vi "KM_fancytorque.vi"() -> ()   [LabVIEW 2016]
uses:
  plot refs -- filter related.ctl
  KM_ControlHFLIcommand.ctl
  cursor winow.ctl
  cursor window action.ctl
  KM_file -- read-write control.ctl
  MQMUser/Documents/Interfaces/Magnet_August_der_Starke.vi
  circle corners.ctl
  lorentzian.ctl
  KM_SystemParameters.ctl
  <vilib>/event_ctls.llb/eventvkey.ctl
  wavepacket.ctl
  filter method control.ctl
  peak -- parameters -- complex fit.ctl
  parameters -- scan monitor control.ctl
panel:
  out "Array of Refnums":refnum<visa-resource-name>[](array[refnum])=["COM3", "16T-Cryocon", "16T-LevelMeter", "16T-Model4G"]
  in  "Update range":bool
  out "Plot: freq vs T":cluster{dbl[], dbl[]}(graph)={[-100.0], [0.0]}
  in  "scan monitor control":T1={"gamma acc. frac. - min "=0.3, "gamma acc frac.. - max"=3.0, "peak acc. fraction (af)"=5.0, "min peak acc. window (kHz)"=0.5, "use"=enum."fraction", "abs gamma min(kHz)"=0.005, "abs gamma max(kHz)"=5.0, "# points"=5, "gamma-factor (fa)"=12.0, "interpolate"=enum."line", "init"=TRUE, "Unique strike parameters"=TRUE, "max peak acc. window (kHz)"=10.0, "spacing factor"=1.5, "iterate #"=1, "overwrite ctl?"=FALSE, "write _m files?"=FALSE, "max slope (kHz/sweep)"=0.5, "funnel state"=enum."funnel open"}
  in  "Plot frequency shift":bool
  in  "Tab : all plot":enum32{"Page 1"}(tab)
  in  "Save frequency scan":path=path "C:/Data/Kim/FancyTorque/YHerb"
  in  "File name":string="lowT_turnonfield"
  in  "ZI HFLI System Parameters IN":T2={"IP Address"="DEV987", "Start (Hz)"=48440.0, "Stop (Hz)"=48480.0, "Filter Order"=4, "Number of Points"=500, "Precision"=0, "Bandwidth (Hz)"=50.0, "Averaging"=1, "Log Sweep"=FALSE, "Demod"=0} {"Averaging" items=["1"=1, "2"=2, "4"=4, "16"=16, "32"=32, "64"=64]; "Bandwidth (Hz)" format="%#_p"; "Precision" items=["Low", "Med", "High"]; "Number of Points" min=2 max=66000; "Filter Order" items=["6, 1st"=1, "12, 2nd"=2, "18, 3rd"=3, "24, 4th"=4, "30, 5th"=5, "36, 6th"=6, "42, 7th"=7, "48, 8th"=8]; "Stop (Hz)" format="%_5p"; "Start (Hz)" format="%_5p"}
  in  "cursor bracket: All, data window":T3={"left"=48455.25, "right "=48459.75, "center"=48457.5, "window"=4.5, "cursors"=[0, 1, 2], "relative"=0, "absolute"=0, "fixed vertical offset"=0.0, "vertical offset"=0.0, "skew"=0.0, "default window frac"=0.1, "kind"=enum."symmetric", "skew.left"=0.5, "skew.right"=0.5, "Plot ref"=refnum, "wing order"=enum."forw"}
  in  "Update system parameters":bool
  out "Plot: All":cluster{"all rows":dbl[], "all rows":dbl[]}[](graph)
  in  "Tab : everything":T4(tab)
  in  "Tab :  Fit controls":enum32{"complex plane", "complex plane 2"}(tab)
  in  "Plot: fragment - filter":cluster{dbl[], dbl[]}[](graph)=[{[], []}, {[], []}, {[], []}, {[], []}]
  in  "scale gauge: Plot: complex plane - filter":dbl(slide)=0.015780000000000002 min=0.0 max=0.3 step=1e-05 scale=0.0001..0.3 scale format="%#_5g"
  in  "Plot: complex plane - filter":cluster{dbl[], dbl[]}[](graph)=[{[], []}, {[], []}, {[0.0, 0.0, 0.0, 0.0, 0.0, 0.0, 0.0, 0.0, 0.0, 0.0, 0.0, 0.0, 0.0, 0.0, 0.0, 0.0, 0.0, 0.0, 0.0, 0.0, 0.0, 0.0, 0.0, 0.0, 0.0, 0.0, 0.0, 0.0, 0.0, 0.0, 0.0, 0.0, 0.0, 0.0, 0.0, 0.0, 0.0, 0.0, 0.0, 0.0, 0.0, 0.0, 0.0, 0.0, 0.0, 0.0, 0.0, 0.0, 0.0, 0.0, 0.0, 0.0, 0.0, 0.0, 0.0, 0.0, 0.0, 0.0, 0.0, 0.0, 0.0, 0.0, 0.0, 0.0, 0.0, 0.0, 0.0, 0.0, 0.0, 0.0, 0.0, 0.0, 0.0, 0.0, 0.0, 0.0, 0.0, 0.0, 0.0, 0.0, 0.0, 0.0, 0.0, 0.0, 0.0, 0.0, 0.0, 0.0, 0.0, 0.0, 0.0, 0.0, 0.0, 0.0, 0.0, 0.0, 0.0, 0.0, 0.0, 0.0], [0.0, 0.0, 0.0, 0.0, 0.0, 0.0, 0.0, 0.0, 0.0, 0.0, 0.0, 0.0, 0.0, 0.0, 0.0, 0.0, 0.0, 0.0, 0.0, 0.0, 0.0, 0.0, 0.0, 0.0, 0.0, 0.0, 0.0, 0.0, 0.0, 0.0, 0.0, 0.0, 0.0, 0.0, 0.0, 0.0, 0.0, 0.0, 0.0, 0.0, 0.0, 0.0, 0.0, 0.0, 0.0, 0.0, 0.0, 0.0, 0.0, 0.0, 0.0, 0.0, 0.0, 0.0, 0.0, 0.0, 0.0, 0.0, 0.0, 0.0, 0.0, 0.0, 0.0, 0.0, 0.0, 0.0, 0.0, 0.0, 0.0, 0.0, 0.0, 0.0, 0.0, 0.0, 0.0, 0.0, 0.0, 0.0, 0.0, 0.0, 0.0, 0.0, 0.0, 0.0, 0.0, 0.0, 0.0, 0.0, 0.0, 0.0, 0.0, 0.0, 0.0, 0.0, 0.0, 0.0, 0.0, 0.0, 0.0, 0.0]}, {[0.0, 0.0, 0.0], [0.0, 0.0, 0.0]}, {[nan, nan, nan, nan, nan, nan, nan, nan, nan, nan, nan, nan, nan, nan, nan, nan, nan, nan, nan, nan], [nan, nan, nan, nan, nan, nan, nan, nan, nan, nan, nan, nan, nan, nan, nan, nan, nan, nan, nan, nan]}, {[0.0, 0.0, 0.0, 0.0, 0.0, 0.0, 0.0, 0.0, 0.0, 0.0, 0.0, 0.0, 0.0, 0.0, 0.0, 0.0, 0.0, 0.0, 0.0, 0.0], [0.0, 0.0, 0.0, 0.0, 0.0, 0.0, 0.0, 0.0, 0.0, 0.0, 0.0, 0.0, 0.0, 0.0, 0.0, 0.0, 0.0, 0.0, 0.0, 0.0]}]
  out "Plot: dz/domega":cluster{"omega out":dbl[], dbl[]}(graph)
  out "Plot: win omega":T5(graph)
  out "Plot: phase":cluster{"omega out":dbl[], dbl[]}(graph)
  out "Plot: phase around center":cluster{dbl[], dbl[]}[](graph)
  out "Plot: fragment":cluster{dbl[], dbl[]}[](graph)
  out "Plot: complex plane":cluster{dbl[], dbl[]}[](graph)=[{[], []}, {[nan, nan, nan, nan, nan, nan, nan, nan, nan, nan, nan, nan, nan, nan, nan, nan, nan, nan, nan, nan, nan, nan, nan, nan, nan, nan, nan, nan, nan, nan, nan, nan, nan, nan, nan, nan, nan, nan, nan, nan, nan, nan, nan, nan, nan, nan, nan, nan, nan, nan], [nan, nan, nan, nan, nan, nan, nan, nan, nan, nan, nan, nan, nan, nan, nan, nan, nan, nan, nan, nan, nan, nan, nan, nan, nan, nan, nan, nan, nan, nan, nan, nan, nan, nan, nan, nan, nan, nan, nan, nan, nan, nan, nan, nan, nan, nan, nan, nan, nan, nan]}, {[nan, nan, nan, nan, nan, nan, nan, nan, nan, nan, nan, nan, nan, nan, nan, nan, nan, nan, nan, nan], [nan, nan, nan, nan, nan, nan, nan, nan, nan, nan, nan, nan, nan, nan, nan, nan, nan, nan, nan, nan]}, {[nan, nan, nan, nan, nan, nan, nan, nan, nan, nan, nan, nan, nan, nan, nan, nan, nan, nan, nan, nan], [nan, nan, nan, nan, nan, nan, nan, nan, nan, nan, nan, nan, nan, nan, nan, nan, nan, nan, nan, nan]}, {[nan, nan, nan, nan, nan, nan, nan, nan, nan, nan, nan, nan, nan, nan, nan, nan, nan, nan, nan, nan], [nan, nan, nan, nan, nan, nan, nan, nan, nan, nan, nan, nan, nan, nan, nan, nan, nan, nan, nan, nan]}, {[nan, nan, nan, nan, nan, nan, nan, nan, nan, nan, nan, nan, nan, nan, nan, nan, nan, nan, nan, nan], [nan, nan, nan, nan, nan, nan, nan, nan, nan, nan, nan, nan, nan, nan, nan, nan, nan, nan, nan, nan]}, {[], []}]
  in  "scale gauge: Plot: complex plane":dbl(slide)=0.013730000000000001 min=0.0 max=0.3 step=1e-05 scale=0.0001..1.0 scale format="%#_2g"
  out "window width (kHz)":dbl=76.27809365793496
  out "window center (kHz)":dbl=3399.029286744401
  out "# of points in window":dbl=953.475933538175
  in  "use fast fit?":bool
  out "pm lorentzian":T6={"Amplitude"=nan, "omega(0)"=0.0, "Gamma"=0.0, "phase"=nan, "Q"=nan, "Norm  Ampl"=nan, "z (inf)"=nan+nani, "4corners"={"z (-pi/2)"=nan+nani, "z(inf)"=nan+nani, "z (pi/2)"=nan+nani, "z center"=nan+nani, "z(0)"=nan+nani, "radius"=nan}} {"z (inf)" format="%#9_9f"; "Q" format="%#9_9f"; "phase" format="%#9_9f"; "Gamma" format="%#9_9f"; "omega(0)" format="%#9_9f"}
  in  "plot staff":enum16{"plot", "do not plot", "a"}(ring)
  in  "Take data":bool=TRUE
  in  "Tab : parameters":enum32{"Page 1"}(tab)
  out "VKey":T8=enum."Return"
  out "Char":i16
  out "Voltage out":cdb[](array[numeric])=[0.0012845876568090215+0.0006495888225572617i, 0.0006617392839354205-0.002163791666582164i, 0.00032146349849778734-0.0008539323430354452i, 0.0007212690079914407-0.0003340132939741794i, 0.0018796838985498537-0.00041382611356276136i, 0.002110516048657634-0.0009455346019583315i, 0.00205017696245498-0.0010893795945051384i, 0.0019478328941950674-0.0014483165844385926i, 0.0018835525878900681-0.001474948715399006i, 0.0013372864726134792-0.0017269565608841629i, 0.0012769136053726307-0.0015682015434732959i, 0.0011465878308944987-0.001449912746741602i, 0.0011207935884417488-0.0014499150090787223i, 0.0012200224050478575-0.001454330158192838i, 0.001088103973473641-0.0013059205845030238i, 0.001072088135514426-0.0012144891963959052i, 0.0011292588329624431-0.0008751147544548225i, 0.0011981393964060746-0.0009880476045942583i, 0.001133057536849098-0.0010263007167294748i, 0.0011273462401748915-0.0011399691730504498i, 0.0012584422806093418-0.0010608947550812256i, 0.0011560305040308565-0.0010341591377315345i, 0.001276567934756488-0.00111907533128109i, 0.0013066630041961857-0.0011064460918718418i, 0.0013770198549916794-0.0010463285175782726i, 0.001314665107953928-0.0009875590410208187i, 0.0013770356718726985-0.0011716715953778503i, 0.0014487115235704165-0.0011144718894301464i, 0.0014447364087279003-0.0012343495924517127i, 0.0014921485718953887-0.0011853078768784987i, 0.0015783944605238338-0.001213834817063661i, 0.0016223257172798958-0.0011418240543088765i, 0.0016368737143736612-0.001111623978754091i, 0.0016204398102554545-0.0010964954268465582i, 0.0016331401454112604-0.0010700307948267869i, 0.0016423618897952804-0.0009410751832895035i, 0.0016255939283663164-0.0009421622662113829i, 0.0016412998435803663-0.0009531512264980333i, 0.0016134375053353611-0.0009005165103711552i, 0.0016054817151254191-0.0009402602111659055i, 0.0015706664673148592-0.0009279919272101116i, 0.0015994002900568897-0.0009699193362076616i, 0.001638610958103286-0.001007835954895566i, 0.001629322361562981-0.0009580956979464267i, 0.0016613871405357136-0.0009785147196610432i, 0.0017233134934095098-0.0009736245027034165i, 0.0016803207109420183-0.0009995146170615366i, 0.0017007833914218493-0.000957625565568956i, 0.0016916365400226811-0.000857954594368348i, 0.0016717789688494263-0.0009179629793560123i, 0.0016734726456965087-0.0009260924684352465i, 0.0017251671295331528-0.000981940013575436i, 0.0017240578858999007-0.0008851005821558551i, 0.001740616055028208-0.0008509351236963866i, 0.0016837038942047505-0.0009158599053328468i, 0.0017068774584739978-0.0008981950544142098i, 0.0017784029248129117-0.0008343945412286558i, 0.0017220291571895204-0.0009102684605824946i, 0.0017414811568882292-0.0008954153399333319i, 0.001791730794309786-0.00086317641219086i, 0.0018095326778530107-0.0008176560683240543i, 0.0018408224973787044-0.0008618058990086667i, 0.001863514774019469-0.0008466857438334946i, 0.0018252400529219098-0.0008819954253651148i, 0.0018496701868752719-0.0008407859865119724i, 0.0017962675417980234-0.0008629872697091864i, 0.0017973106898536751-0.0007803741540721287i, 0.0018817654775391502-0.0008525743688557984i, 0.0019151590883315485-0.0007186850689094861i, 0.0018794337717190372-0.0008764653298521186i, 0.0019260508004357265-0.0007941075642398263i, 0.0018776042728789616-0.0007661555133994668i, 0.0019143345542945859-0.0007753066474220565i, 0.0019737687259583575-0.0008375058894921223i, 0.0019540134386967127-0.0007637184747032095i, 0.0019582567995273252-0.0007733951871243031i, 0.001953782904316904-0.0007086374682689142i, 0.0019816663652331328-0.0007333547766448622i, 0.0019937754726138154-0.0007473992751162255i, 0.0020231747092911883-0.0007664609443880946i, 0.0020039630201527225-0.00070309945416075i, 0.002026570187391667-0.0006924798114057269i, 0.0020517692852400765-0.0007059972645268008i, 0.002111150248456159-0.0007383014760781856i, 0.0020888694840294248-0.0006867111807744941i, 0.002107977724150776-0.0006963636892461208i, 0.0021037562899836448-0.0006685917995638402i, 0.0022056155979483572-0.0006809342679433687i, 0.002097789981748124-0.0006425438747908021i, 0.0021469903646535366-0.0006385474701970675i, 0.002150326224640565-0.0006426478060220725i, 0.002242371255515889-0.0006443963159867091i, 0.0021873894789702147-0.000634045662812584i, 0.0022957618136050196-0.0005750313735194432i, 0.002253170671362487-0.0005832140414506337i, 0.0023235996015851775-0.0006057693151380434i, 0.0023016412783703403-0.0005390881913130007i, 0.002279165717468865-0.0005042541103480928i, 0.002336740876626925-0.0005380171670209624i, 0.00233171734153575-0.0005790701993690402i, 0.002388427065202294-0.0004847594462102123i, 0.0024078618617769713-0.0005321359610903262i, 0.0024050254670876783-0.0004724195462420472i, 0.0023880577604300517-0.0004817079305537639i, 0.0024496700333396315-0.0003755508762008526i, 0.002438976677805125-0.00046093380231800496i, 0.002493137702980762-0.00041814856498941275i, 0.002492956546968145-0.0004336085229735855i, 0.002553550885423945-0.0004259610679846094i, 0.0025692366701788334-0.0003384157924222541i, 0.0026110322949625168-0.0004042061129842982i, 0.002594048021942123-0.00038038382050690074i, 0.0026935057630560425-0.00032149661348098216i, 0.002611293396751969-0.0003410715034981749i, 0.0026791494396341494-0.00025413015786752014i, 0.002709640921499399-0.00028845444266075506i, 0.002778407060136788-0.0002918891245380796i, 0.0027451063419710975-0.0002232337565398509i, 0.002784644881819971-0.0002510748836284296i, 0.0027907520982866675-0.00020485080622197063i, 0.0029181356584552466-0.00023917410861805518i, 0.002812255052563042-0.0002205159302104745i, 0.0029056009833786475-0.0001857379925028191i, 0.0029549266152767966-0.00019850956081394526i, 0.0029519250295100717-8.865159284196847e-05i, 0.0030038798266967706-0.00016557378499429463i, 0.00307375138145389-3.792811670582832e-05i, 0.0030359615585887887-8.441794575385311e-05i, 0.003129281247803782-4.6591584464395374e-05i, 0.003119498942335888-4.790723055434046e-05i, 0.003156268492608772+3.3369060301053233e-06i, 0.0031604717877623026-3.238527041469325e-05i, 0.0032182645504561544+7.175506943461175e-05i, 0.00325157439422464+6.360385776655813e-05i, 0.0032312536208319864+6.841236181026814e-05i, 0.003327834859828407+0.00011397821319413468i, 0.003352054093981589+0.00013870101558009177i, 0.0035022320352406594+0.00019252256901124552i, 0.003460365402365128+0.0001941569994280293i, 0.0035431052575024954+0.0002484850455581141i, 0.003614690194051692+0.0002469419701488894i, 0.003632986127779432+0.00026591742334990695i, 0.0035951409257101953+0.0003299427555412546i, 0.0036791434452897753+0.0003945573282901271i, 0.0037680957686082144+0.0004095717015192001i, 0.0038267326807418303+0.00041677933808913236i, 0.00379277892041235+0.000510023078536785i, 0.003981975247219429+0.000567566514919109i, 0.003979461191138457+0.0006118795104304059i, 0.004095449787916228+0.0005678155014081981i, 0.004082532679037655+0.0006789879733919079i, 0.0041416705169278496+0.0006968975155678261i, 0.0041752270356982465+0.0007417221199894664i, 0.004306741887394477+0.0007047938316415208i, 0.004381171768553447+0.0007614265187465232i, 0.004410861470593261+0.0008429185780512395i, 0.00440183077633223+0.0008604872336254198i, 0.004561085055645665+0.0009675595013794393i, 0.004552727745330181+0.0009970456097637577i, 0.00471663770122752+0.0011496926933133908i, 0.004796223280094124+0.0011597629642857447i, 0.004933398880461905+0.0011462201339557728i, 0.004929032038379632+0.001264843652165741i, 0.005041034391262139+0.0013742509765506889i, 0.00517115251414733+0.0014281603482237616i, 0.0052184702074318185+0.0014480939145209398i, 0.005382800183939043+0.001487143234254288i, 0.005434423140701515+0.0016735209038047918i, 0.005628787852046442+0.0017763135558037891i, 0.005708963960394959+0.001828463918501302i, 0.005807834872097633+0.001955157602426399i, 0.005954152301800823+0.0020309652402478126i, 0.006071519887993931+0.002207640738931057i, 0.006202919659851819+0.002302726532472194i, 0.006378519683105122+0.0024202392805281613i, 0.006501213424462855+0.0025043431301609437i, 0.00665272340029824+0.0026777718654535623i, 0.006885223229515294+0.0029258478128129i, 0.007079466259436847+0.003002977370340245i, 0.007225697740487776+0.003136437586511814i, 0.007411093295179831+0.003348180576308869i, 0.007562960518093076+0.003551323080106507i, 0.007839319171981673+0.003755237524359879i, 0.008003012941616452+0.003965478762243461i, 0.008242690897210771+0.004183777336771237i, 0.008507865454515538+0.004474962342874131i, 0.008808283140172945+0.00477281568658155i, 0.00908058916905025+0.005121249957065217i, 0.00935987768948563+0.00546204505815727i, 0.009690951524422436+0.005811341689045154i, 0.010041275063688761+0.006243502419167194i, 0.010377308661253215+0.0066814428850399295i, 0.010821090442537928+0.007246326014229916i, 0.01110339104405149+0.007763749750973363i, 0.011548922285157782+0.008437832276552346i, 0.011938534912557083+0.009147998559390448i, 0.012402554738703681+0.010027270519608483i, 0.012829242375072745+0.010923908915455327i, 0.013265063889717339+0.011892897004622314i, 0.01366229812717843+0.013158590460522883i, 0.014148688473608227+0.014497482157698239i, 0.014556072459345228+0.016225206473959836i, 0.014867277607117415+0.017880934985240904i, 0.015017026872222571+0.019957728269853706i, 0.015032475553930322+0.022276251021974475i, 0.01474431220463535+0.02497837480891795i, 0.014167833693749457+0.02777077756959768i, 0.013181912865208352+0.031193625409082645i, 0.011385283493448252+0.03489812886044834i, 0.008957576161982015+0.038715216070463146i, 0.005242329278194911+0.0427968401413087i, 0.0006252278100432423+0.04661593281159648i, -0.005911287732882362+0.05011026344278879i, -0.013591238426411825+0.05251628172902849i, -0.02337790721019255+0.0534413622856662i, -0.033630245398644704+0.05188020627236112i, -0.045305810931312925+0.0471735714866712i, -0.05629251580669748+0.03843226912802993i, -0.06452110462180362+0.026700916103135557i, -0.06948912856925225+0.011212410316730072i, -0.06899893101144594-0.005780785783534742i, -0.06261013071656525-0.021705049812832784i, -0.05100184594823542-0.03419481076161618i, -0.032946350042392304-0.041571415418816794i, -0.01868668431448581-0.04087977118020359i, -0.005543822677633614-0.034517566998955265i, 0.002818039193472556-0.024763983161266937i, 0.0061020718520623475-0.012426604308897724i, 0.003800347891064826-0.001572543758658912i, -0.002848933816338246+0.006190187019292026i, -0.012604222470420806+0.008955874209654479i, -0.02155552822317469+0.005238325471119359i, -0.02589544941540957-0.0026208465243363352i, -0.024475689744310636-0.011436477784249216i, -0.017189384940711688-0.01770822527519569i, -0.008529115283883103-0.017806247487492086i, -0.0020597678425682653-0.01259062840821534i, -0.0007919835493477994-0.005017709121603978i, -0.005247590304852724+0.0008351545385979753i, -0.01159992036923221+0.0012133469390995454i, -0.015541311327444544-0.003410449836750198i, -0.014282943396979945-0.00918833467586662i, -0.008553779761081463-0.011838183938914048i, -0.0036128749788524473-0.009032305153930546i, -0.0030516232692530403-0.0038885885290287432i, -0.006986413581267574-0.0009127950863942365i, -0.010797787706180284-0.002856690243270585i, -0.010641437801974265-0.006984007270417016i, -0.006515514154564542-0.008743162630022639i, -0.003584326419135037-0.006190693631128883i, -0.004751762804060355-0.0026018979981187553i, -0.008042694130786317-0.0028808846691022443i, -0.008578872913754244-0.005739785681268362i, -0.00565505072285471-0.0070802542585224225i, -0.0037522014079977113-0.005046225793730637i, -0.005086702938481904-0.0028817844511973604i, -0.007192865067067861-0.00372018477856524i, -0.006423967248421029-0.005912268622839845i, -0.004284382561999433-0.005525437290348685i, -0.004218903549595074-0.0035773538394296743i, -0.005878373648998807-0.0034656559274377136i, -0.005920773294388874-0.005072802421290534i, -0.004186379168512512-0.005105039767095756i, -0.004085196644076723-0.0036503674101985004i, -0.005265859755533027-0.0035820414151557264i, -0.005108048724465077-0.004825906468732111i, -0.0039049456628715094-0.00443047123163233i, -0.004189142064462894-0.0034511589351929883i, -0.00500467804446355-0.003931426194746052i, -0.004160442694023512-0.004630699642880589i, -0.003728008962588712-0.0038130079921045675i, -0.004407974342097486-0.0035870227018844816i, -0.004272395514897711-0.004344656769900021i, -0.003639110575984402-0.003889317942454068i, -0.00402715242953899-0.003486845612159572i, -0.004169957988068188-0.004050105083553233i, -0.003537455555438435-0.0038858913604457785i, -0.0037730415518572907-0.0034867848996079807i, -0.003942125201253654-0.003852739380319232i, -0.003428914546716074-0.003830177912139123i, -0.003580483612622666-0.003518430370457909i, -0.003634267043729232-0.0038741155177839932i, -0.0033080633540293614-0.0036867298525101793i, -0.0035040116919212213-0.0034748256693246807i, -0.003427766201305557-0.003718309633742351i, -0.0031887492219475557-0.0035270824550330177i, -0.003372230379493813-0.003582833850732337i, -0.0032443254974273868-0.0035692200033260986i, -0.0031717344327815565-0.003320021154204544i, -0.00316470134610925-0.0035859789955868587i, -0.0030544039668105624-0.0034508963387435i, -0.00310526168700391-0.0034612342602408142i, -0.0029289045124791502-0.0034670060690914174i, -0.002929996742265166-0.0034312918223401868i, -0.0029794201349106703-0.003502071136299563i, -0.002861255585975232-0.003358983590000057i, -0.0029525709433300745-0.003408372313357868i, -0.002704827015705849-0.003374363087453031i, -0.002849301996246121-0.0032811601136936456i, -0.0027632284160914932-0.0033104866711017255i, -0.00274594009100205-0.0031633873874291046i, -0.0026970152868806786-0.0032626649782568472i, -0.0026213977094616697-0.0032539243890000033i, -0.002579561026486845-0.0032564634439627813i, -0.0025928100781667227-0.0032070620108229616i, -0.002550092697588366-0.0032548413967179476i, -0.0024987582956025457-0.003172052964638669i, -0.002521446727213947-0.003202944659716233i, -0.002520178823496431-0.003162011975851037i, -0.0024232508019298845-0.003114243875820886i, -0.002446579589252357-0.0031933203387646885i, -0.00240421131088523-0.0031306314897205827i, -0.0023928775624939874-0.0031027562256900148i, -0.002322391452257384-0.0031116843878731715i, -0.0023424802056701112-0.00314544547869475i, -0.002225603021005885-0.0030756389281725613i, -0.0022052266501405627-0.003070435681748255i, -0.002254471057454397-0.003043314223840779i, -0.0022266417195091195-0.0030649446105502215i, -0.0022500042283008235-0.0030229615258627073i, -0.0021531914460271827-0.002958959927864058i, -0.0021493964487041385-0.002964426146799965i, -0.002140406584852801-0.0030376290981753195i, -0.0021117867789186883-0.0030719295906413797i, -0.0020963292856098132-0.0029896691253815896i, -0.0021127200261628447-0.002987393477504498i, -0.0020620405926304614-0.002901284688695035i, -0.0020482598662084966-0.002964298656383419i, -0.002029445821946481-0.002867706094527497i, -0.002010154424250043-0.002940876524797307i, -0.0020078701098060208-0.002907163167439238i, -0.0019167565524693306-0.0029384817261585445i, -0.0020066163491496017-0.0028921513333277924i, -0.0019026631777767523-0.0028566600904277066i, -0.001882355287588045-0.0028059822173907662i, -0.0019091487232228994-0.0028806750669088752i, -0.0018670193817058906-0.0028720585731661584i, -0.0019052465095421777-0.0028718189239799576i, -0.001811093484202012-0.0028156065148620224i, -0.001810705585381768-0.0028685516449326407i, -0.0018816429965024793-0.002838603854960726i, -0.0018275653909028853-0.0028352821560036325i, -0.0017990893881458705-0.0027910293638010145i, -0.001786574494948073-0.002798058569053285i, -0.0017665843339077095-0.0027787166598958624i, -0.0017258679993081033-0.002766553630598918i, -0.0016870144906848566-0.0027382849504088073i, -0.0016806434217619863-0.0027836065615683297i, -0.001611539048209973-0.0027789827820880906i, -0.0015878562684343224-0.0027729675656951425i, -0.001668724204230745-0.0027324238763718196i, -0.001630593035350544-0.0027828853361952454i, -0.0016662708043788717-0.002777578180056975i, -0.0016248172089546318-0.0027272042193398427i, -0.0015960009193624763-0.0026907990577764856i, -0.0016484655286512044-0.002696460951848219i, -0.001618902841835217-0.0027971632038948807i, -0.0016024448758572634-0.002731856683352187i, -0.0016162466849358123-0.002689238611408242i, -0.0015624343486881286-0.0026975115987983196i, -0.0015435241424523558-0.002714551170163077i, -0.0015085982020689329-0.002732647805769127i, -0.0015140047175016586-0.002675825035838422i, -0.0014874007277802443-0.0026815290681945665i, -0.0014082664048756532-0.002643098148894566i, -0.0015073342504388154-0.002683875424959701i, -0.0014254436772604773-0.002644687782242889i, -0.0015013972967163646-0.0026679540930476604i, -0.0014536795661329776-0.002663653264550726i, -0.0014501132330715883-0.0026176690219077963i, -0.0014308230390608074-0.0026848828107240057i, -0.0013498915119992251-0.0026707013666032713i, -0.0014384716376379819-0.002652145578636841i, -0.0013808433340556554-0.0026682805919705046i, -0.0013939586990143053-0.0026060937246164652i, -0.0014003464458879377-0.0026316687458094964i, -0.0014029460978128485-0.002566058047793383i, -0.0013261118836590021-0.0026698574995309638i, -0.001328134134301238-0.002638543175795008i, -0.001305358076140691-0.0025771236500066303i, -0.0013403184399105226-0.0025613522564219204i, -0.0013547281618873927-0.002603713614898883i, -0.0013676523549426504-0.0025787908605671254i, -0.0013363824351501964-0.0026323379977527656i, -0.0013313580263053923-0.0026298374931202195i, -0.0013110506222568056-0.002573221194048591i, -0.0012330165359166038-0.0025477892830999i, -0.001274819429850306-0.0025776032022077457i, -0.0012913249699882039-0.002559903111000059i, -0.0012351958759552527-0.0025531513867371944i, -0.0012080508556160307-0.0024967977422495303i, -0.001242890936964886-0.002516181533824169i, -0.0011911832365192993-0.002537438522641241i, -0.0012117460659409724-0.002531880096612451i, -0.0011775131862113456-0.002479508235520232i, -0.0011697723985856254-0.0025245200031333752i, -0.00125285962118635-0.002502058742256083i, -0.0011924658842724987-0.002545556621666579i, -0.001175867208475582-0.002496083291581419i, -0.00115324279107653-0.0024854896736684596i, -0.0012424790032381523-0.0025229966419555616i, -0.0012061607462239448-0.0024999218126768937i, -0.00120868989937542-0.0024713945826498425i, -0.0011737551729851428-0.0024557837321779337i, -0.0012022616076305223-0.0025043760446179448i, -0.0011450136011439175-0.002469479480868892i, -0.0012256798439802235-0.002490653753386086i, -0.0011739597308424521-0.0024865224102169i, -0.0011485280818009016-0.002408525987995914i, -0.0011629508030996719-0.0024865504049117193i, -0.0010955285363504657-0.0024828137624475053i, -0.0011234513041756113-0.0024813917404583117i, -0.0011862510289539308-0.0024744193445937926i, -0.001156313967208874-0.0024747145709433454i, -0.0011036037861897959-0.002467676937399998i, -0.001162771297351189-0.002511495985707852i, -0.0012109454639804256-0.0024655211428812472i, -0.0011606536283279975-0.0024822913388635823i, -0.0010967451125348487-0.0025180901501380415i, -0.0010719574294308476-0.0024843711715536094i, -0.0010659702183026237-0.00249804687819511i, -0.001055127638060358-0.0025139187661310505i, -0.000959779420812176-0.0024636980793767012i, -0.0010421155618337663-0.0024208184996079613i, -0.0010033315103198386-0.002434326503762653i, -0.0010048686835697309-0.0024687943021930933i, -0.001002035846030894-0.002466917828506675i, -0.0009753937011426879-0.0024121584444941526i, -0.0009798258868293352-0.0023625261501379687i, -0.0009669245495321893-0.002441961010014273i, -0.0010215000017995992-0.002462411354584728i, -0.0009708259996127895-0.00241439997936254i, -0.0010085818571458566-0.0024837085325957694i, -0.0009352128046242682-0.002394666113145431i, -0.0009027192004619631-0.002370381853089013i, -0.0009759951587736593-0.0023629132185411933i, -0.0009243352296922402-0.002354215121283074i, -0.000918581060653735-0.0023798754025745683i, -0.0009947541256023213-0.002358947269165113i, -0.0009135780204569385-0.0024080207165739814i, -0.0009996556860307642-0.002410421137420598i, -0.0009246854062587925-0.0023627119908078854i, -0.0009185395312713385-0.0024283055861140626i, -0.0009736557858466129-0.0023975500810886766i, -0.0009424947678586537-0.0024145452580983454i, -0.0009440465547569038-0.00240429251946369i, -0.0009415765612115092-0.0023495610860543837i, -0.0009498653020631775-0.002360027056965208i, -0.0008761482284051203-0.002420634784923393i, -0.0008582745250013607-0.0023173095601178987i, -0.0009088686504932125-0.002333561310273478i, -0.0008992079946634785-0.0023350284631136254i, -0.0008797040193454746-0.0023164268867726643i, -0.0009224217512221669-0.0023835391577688627i, -0.0008825546954861182-0.002350405914988027i, -0.0008818456714826222-0.0023715896052903837i, -0.0008228708233361892-0.002316090386605913i, -0.0008643934015830207-0.0023458754807529187i, -0.0008494570683769504-0.002410604176008757i, -0.0008391115564800117-0.002398368587637436i, -0.0008093905767329528-0.002392350889808341i, -0.0008577846258449522-0.002317396705434379i, -0.000810653711007433-0.002325267804055737i, -0.0008486063667287098-0.002361332598377178i, -0.0008701445483082514-0.0023232791411734372i, -0.0008408228691377277-0.002360253132581682i, -0.0008198193079062388-0.0023501085145600587i, -0.0007879367492600357-0.0022598307809756314i, -0.000835439115617459-0.002343027253055219i, -0.0008056869165996285-0.002313292504572691i, -0.0008523203259507584-0.0022949487146195478i, -0.000754547128002699-0.002413636829670117i, -0.000753764451468177-0.0023065690428762326i, -0.0008153735451013964-0.0022953778905789608i, -0.0007629800835782574-0.002345037392474055i, -0.0008176576546402645-0.0023130804864765846i, -0.0007393740416888393-0.0022865787953136483i, -0.0008197160806306269-0.002264098983800463i, -0.0007934252041046379-0.0023085780255699883i, -0.0007827998985231264-0.00230619406991705i, -0.0007396252402325018-0.002299798869977056i, -0.0007984543469832971-0.0023459015245453118i, -0.00073803554014278-0.0022384644668783796i, -0.0007972271623139771-0.002297631864866292i, -0.0007574875862735704-0.00232073209113468i, -0.0007167160970048067-0.002341009000026472i, -0.0007285857191083117-0.0022924795178939756i, -0.00072819190650184-0.0022831559247009263i, -0.0006664511366187818-0.002304097317678437i, -0.0007213001307740816-0.0022811048288640325i, -0.0007106707771455356-0.002303140516080962i, -0.0007655095548083673-0.002272989447134717i, -0.0007259711620321689-0.0022856077807427064i, -0.0007008895156067375-0.002308652646681789i, -0.0007287060253870731-0.0022381151242018152i, -0.0007340181303547636-0.0022588461358329756i, -0.0008073883845990267-0.0022241967100476642i, -0.0006777450584392889-0.002309375982487362i, -0.0006849974006480055-0.002273180023725972i, -0.0007249970026880554-0.0022813185273485017i]
  out "Freq out":dbl[](array[numeric])=[48439.99999999998, 48440.08012730833, 48440.16025474932, 48440.24038232274, 48440.32051002872, 48440.40063786724, 48440.4807658384, 48440.560893942005, 48440.64102217816, 48440.72115054695, 48440.801279048195, 48440.88140768198, 48440.96153644841, 48441.041665347286, 48441.121794378705, 48441.20192354268, 48441.28205283929, 48441.36218226835, 48441.44231182996, 48441.52244152421, 48441.60257135091, 48441.68270131016, 48441.762831402055, 48441.8429616264, 48441.923091983284, 48442.003222472726, 48442.083353094815, 48442.16348384935, 48442.243614736435, 48442.32374575616, 48442.40387690835, 48442.48400819308, 48442.56413961046, 48442.644271160294, 48442.72440284267, 48442.80453465761, 48442.88466660519, 48442.96479868522, 48443.044930897806, 48443.12506324304, 48443.20519572073, 48443.28532833097, 48443.36546107385, 48443.445593949196, 48443.525726957094, 48443.60586009754, 48443.68599337064, 48443.766126776194, 48443.8462603143, 48443.92639398506, 48444.00652778827, 48444.08666172403, 48444.16679579245, 48444.24692999333, 48444.32706432676, 48444.40719879274, 48444.48733339138, 48444.56746812247, 48444.64760298612, 48444.72773798243, 48444.80787311119, 48444.8880083725, 48444.96814376648, 48445.0482792929, 48445.12841495189, 48445.20855074343, 48445.288686667634, 48445.36882272429, 48445.448958913505, 48445.529095235375, 48445.609231689705, 48445.689368276595, 48445.76950499604, 48445.849641848145, 48445.92977883271, 48446.009915949835, 48446.090053199616, 48446.170190581855, 48446.25032809666, 48446.33046574412, 48446.41060352404, 48446.49074143652, 48446.570879481565, 48446.65101765927, 48446.731155969435, 48446.81129441216, 48446.89143298755, 48446.9715716954, 48447.05171053581, 48447.13184950888, 48447.211988614414, 48447.29212785252, 48447.372267223174, 48447.4524067265, 48447.53254636229, 48447.61268613064, 48447.69282603165, 48447.77296606513, 48447.853106231174, 48447.93324652988, 48448.01338696105, 48448.09352752478, 48448.17366822108, 48448.25380905005, 48448.33395001148, 48448.41409110548, 48448.494232332145, 48448.57437369127, 48448.65451518296, 48448.734656807326, 48448.814798564155, 48448.89494045355, 48448.97508247552, 48449.055224630145, 48449.13536691724, 48449.21550933691, 48449.29565188924, 48449.37579457404, 48449.45593739141, 48449.53608034145, 48449.61622342396, 48449.69636663904, 48449.77650998668, 48449.856653466995, 48449.93679707978, 48450.01694082514, 48450.097084703164, 48450.17722871366, 48450.25737285673, 48450.337517132466, 48450.417661540676, 48450.497806081454, 48450.57795075481, 48450.65809556083, 48450.738240499326, 48450.8183855704, 48450.89853077414, 48450.97867611035, 48451.058821579136, 48451.138967180596, 48451.21911291453, 48451.29925878104, 48451.37940478011, 48451.459550911866, 48451.53969717609, 48451.619843572895, 48451.699990102374, 48451.780136764326, 48451.86028355885, 48451.940430485956, 48452.020577545736, 48452.10072473799, 48452.18087206282, 48452.26101952032, 48452.3411671103, 48452.42131483286, 48452.501462688095, 48452.58161067581, 48452.6617587961, 48452.74190704896, 48452.82205543451, 48452.90220395254, 48452.98235260313, 48453.06250138641, 48453.14265030217, 48453.22279935051, 48453.30294853152, 48453.38309784502, 48453.463247291096, 48453.54339686975, 48453.62354658108, 48453.70369642489, 48453.78384640129, 48453.863996510365, 48453.94414675192, 48454.02429712605, 48454.104447632875, 48454.18459827217, 48454.26474904405, 48454.34489994852, 48454.42505098566, 48454.50520215529, 48454.5853534575, 48454.66550489239, 48454.74565645977, 48454.82580815972, 48454.905959992364, 48454.98611195749, 48455.066264055204, 48455.1464162855, 48455.226568648475, 48455.306721143934, 48455.38687377198, 48455.467026532715, 48455.54717942593, 48455.62733245173, 48455.70748561022, 48455.787638901194, 48455.86779232475, 48455.9479458809, 48456.02809956973, 48456.10825339105, 48456.18840734496, 48456.26856143155, 48456.34871565063, 48456.4288700023, 48456.50902448666, 48456.5891791035, 48456.66933385294, 48456.74948873495, 48456.82964374966, 48456.909798896864, 48456.98995417665, 48457.07010958913, 48457.15026513409, 48457.23042081165, 48457.31057662179, 48457.39073256463, 48457.47088863995, 48457.551044847874, 48457.63120118848, 48457.71135766158, 48457.79151426727, 48457.871671005654, 48457.951827876524, 48458.03198487999, 48458.11214201605, 48458.1922992848, 48458.27245668604, 48458.35261421988, 48458.43277188641, 48458.51292968543, 48458.593087617046, 48458.673245681355, 48458.75340387816, 48458.833562207554, 48458.913720669545, 48458.993879264235, 48459.07403799141, 48459.15419685119, 48459.23435584366, 48459.31451496863, 48459.39467422619, 48459.47483361645, 48459.5549931392, 48459.63515279455, 48459.715312582506, 48459.795472503145, 48459.875632556286, 48459.955792742025, 48460.03595306046, 48460.116113511394, 48460.196274094924, 48460.27643481115, 48460.35659565988, 48460.43675664121, 48460.516917755136, 48460.59707900176, 48460.677240380886, 48460.7574018926, 48460.837563537025, 48460.91772531395, 48460.99788722347, 48461.07804926569, 48461.158211440415, 48461.23837374774, 48461.31853618767, 48461.39869876029, 48461.47886146542, 48461.55902430315, 48461.63918727358, 48461.71935037651, 48461.799513612044, 48461.87967698029, 48461.959840481024, 48462.040004114366, 48462.12016788031, 48462.200331778964, 48462.28049581012, 48462.36065997387, 48462.440824270336, 48462.520988699296, 48462.60115326087, 48462.68131795515, 48462.76148278192, 48462.841647741305, 48462.921812833294, 48463.00197805799, 48463.082143415195, 48463.162308905, 48463.24247452751, 48463.32264028253, 48463.40280617016, 48463.482972190395, 48463.563138343336, 48463.64330462878, 48463.72347104683, 48463.8036375976, 48463.88380428087, 48463.963971096746, 48464.044138045334, 48464.12430512643, 48464.204472340134, 48464.28463968645, 48464.364807165475, 48464.444974777005, 48464.525142521146, 48464.605310398, 48464.685478407366, 48464.765646549335, 48464.84581482402, 48464.92598323122, 48465.00615177102, 48465.086320443435, 48465.166489248564, 48465.2466581862, 48465.32682725646, 48465.406996459424, 48465.4871657949, 48465.56733526299, 48465.64750486379, 48465.7276745971, 48465.80784446303, 48465.88801446157, 48465.96818459283, 48466.0483548566, 48466.12852525298, 48466.20869578207, 48466.28886644369, 48466.36903723791, 48466.44920816486, 48466.52937922431, 48466.60955041638, 48466.68972174107, 48466.76989319848, 48466.8500647884, 48466.93023651093, 48467.010408366186, 48467.09058035396, 48467.17075247434, 48467.25092472744, 48467.33109711306, 48467.4112696313, 48467.49144228216, 48467.57161506573, 48467.65178798183, 48467.73196103054, 48467.81213421197, 48467.892307525915, 48467.97248097249, 48468.05265455177, 48468.13282826358, 48468.21300210801, 48468.293176085055, 48468.37335019482, 48468.45352443711, 48468.53369881202, 48468.61387331964, 48468.6940479598, 48468.774222732565, 48468.85439763796, 48468.93457267607, 48469.01474784671, 48469.09492314997, 48469.175098585954, 48469.25527415446, 48469.335449855585, 48469.415625689435, 48469.49580165581, 48469.57597775481, 48469.65615398643, 48469.736330350774, 48469.816506847645, 48469.896683477135, 48469.97686023935, 48470.057037134095, 48470.13721416146, 48470.21739132156, 48470.29756861418, 48470.37774603942, 48470.45792359729, 48470.538101287886, 48470.61827911101, 48470.69845706676, 48470.778635155235, 48470.85881337624, 48470.938991729876, 48471.019170216234, 48471.099348835116, 48471.17952758663, 48471.25970647077, 48471.33988548764, 48471.420064637045, 48471.50024391907, 48471.58042333383, 48471.660602881115, 48471.74078256103, 48471.82096237368, 48471.90114231885, 48471.981322396656, 48472.061502607095, 48472.14168295026, 48472.221863425955, 48472.30204403429, 48472.38222477534, 48472.462405648934, 48472.54258665516, 48472.62276779411, 48472.7029490656, 48472.78313046972, 48472.86331200647, 48472.94349367595, 48473.02367547797, 48473.10385741262, 48473.18403948, 48473.26422167992, 48473.344404012474, 48473.424586477755, 48473.504769075575, 48473.58495180603, 48473.66513466912, 48473.74531766494, 48473.825500793304, 48473.9056840543, 48473.98586744803, 48474.066050974296, 48474.1462346332, 48474.226418424834, 48474.306602349, 48474.38678640582, 48474.46697059527, 48474.547154917454, 48474.62733937217, 48474.707523959536, 48474.78770867963, 48474.86789353227, 48474.94807851754, 48475.02826363545, 48475.10844888611, 48475.188634269296, 48475.268819785124, 48475.349005433694, 48475.429191214804, 48475.509377128554, 48475.58956317504, 48475.66974935407, 48475.749935665735, 48475.83012211005, 48475.9103086871, 48475.99049539669, 48476.07068223892, 48476.150869213896, 48476.23105632141, 48476.31124356157, 48476.39143093447, 48476.471618439915, 48476.551806077994, 48476.63199384873, 48476.7121817522, 48476.79236978821, 48476.87255795687, 48476.95274625827, 48477.032934692215, 48477.11312325881, 48477.19331195814, 48477.27350079002, 48477.35368975454, 48477.43387885171, 48477.514068081626, 48477.594257444085, 48477.67444693919, 48477.75463656704, 48477.83482632744, 48477.91501622048, 48477.99520624627, 48478.07539640461, 48478.15558669559, 48478.235777119226, 48478.315967675604, 48478.39615836453, 48478.4763491861, 48478.556540140424, 48478.63673122729, 48478.716922446816, 48478.79711379908, 48478.877305283895, 48478.95749690136, 48479.03768865148, 48479.117880534344, 48479.19807254976, 48479.27826469782, 48479.35845697864, 48479.438649392, 48479.51884193802, 48479.59903461679, 48479.67922742811, 48479.75942037208, 48479.839613448705, 48479.91980665807, 48480.0]
  in  "parameters: complex fit":T9={"main VI path"=path "", "scale factor"=3.0, "# of grid points"=200, "parameters: wavepacket"={"R"=0.5, "wave number"=22.0, "delta k"=7.0, "radii vector"=[], "radial section"=[], "wave vector"=22.0, "wavepacket is"=TRUE}, "span"=0.27789, "interference ?"=enum."cp z center", "filter method"=enum."three"} {"span" min=0.0 max=0.5 step=1e-05 scale=0.0001..0.5 scale format="%#_5f"; "parameters: wavepacket"."delta k" format="%#_3f"; "parameters: wavepacket"."wave number" format="%#_3f"; "parameters: wavepacket"."R" format="%#_3f"}
  # "three strikes"
  # "search window"
  # "linear extrapolation"
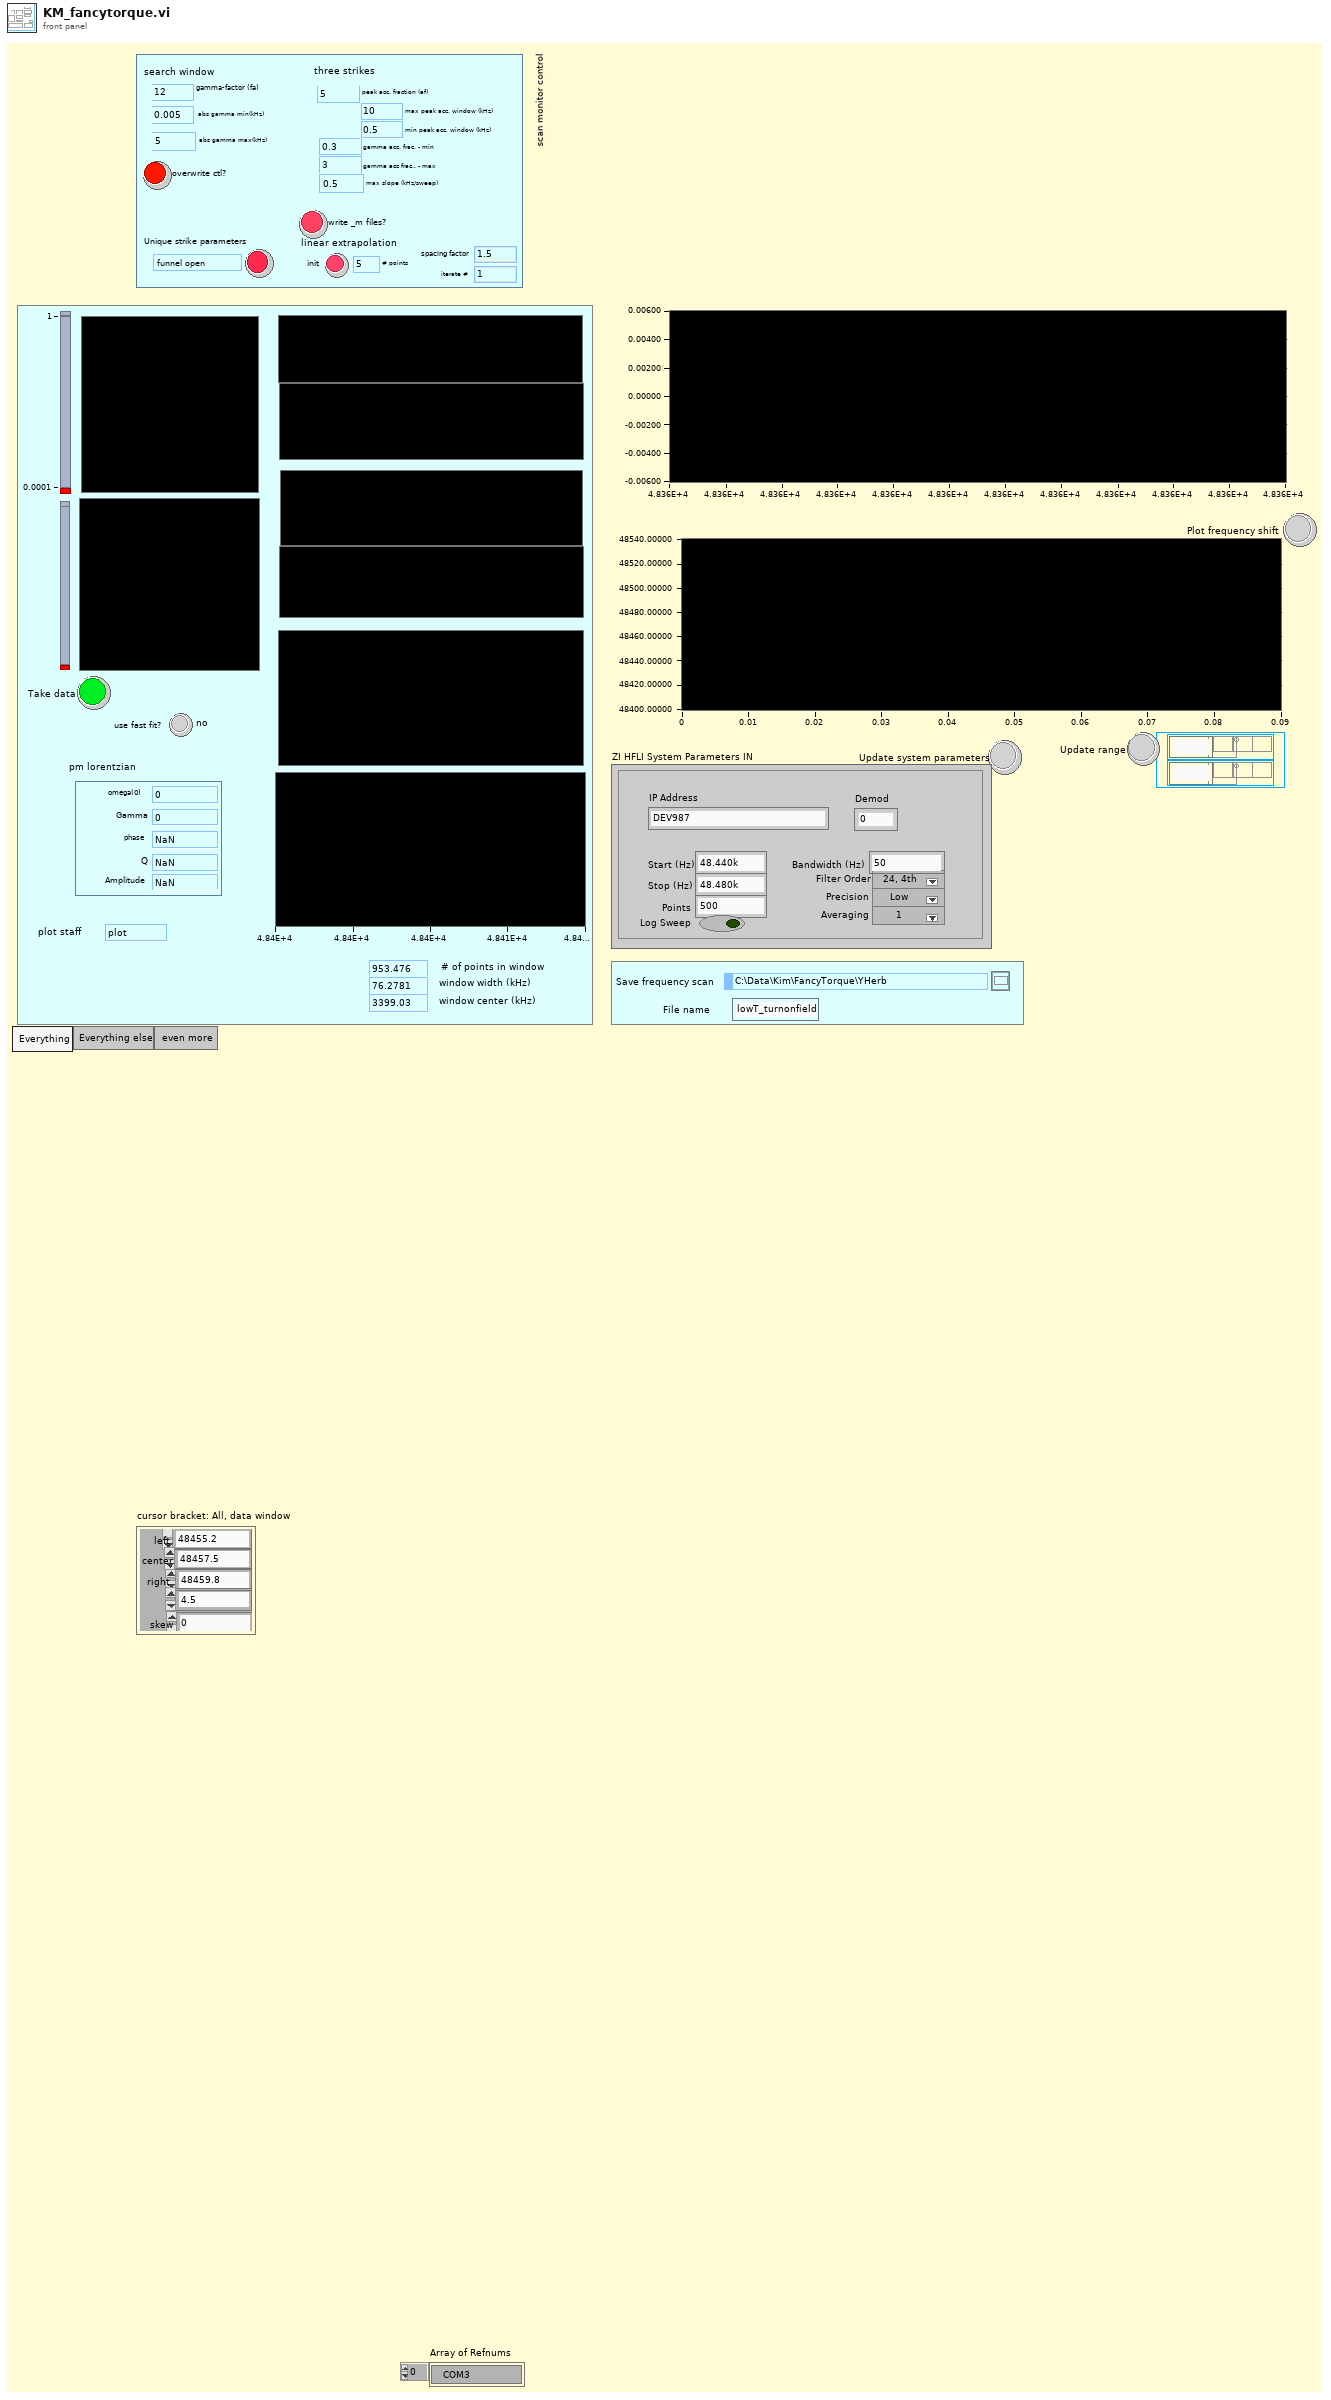
[diagram p1: front panel]
types:
  T1 = typedef "parameters -- scan monitor control.ctl" = cluster{"gamma acc. frac. - min ":dbl, "gamma acc frac.. - max":dbl, "peak acc. fraction (af)":dbl, "min peak acc. window (kHz)":dbl, "use":enum16{"window", "fraction"}, "abs gamma min(kHz)":dbl, "abs gamma max(kHz)":dbl, "# points":i32, "gamma-factor (fa)":dbl, "interpolate":enum16{"line", "last"}, "init":bool, "Unique strike parameters":bool, "max peak acc. window (kHz)":dbl, "spacing factor":dbl, "iterate #":i32, "overwrite ctl?":bool, "write _m files?":bool, "max slope (kHz/sweep)":dbl, "funnel state":enum16{"funnel open", "funnel closed"}}
  T2 = typedef "KM_SystemParameters.ctl" = cluster{"IP Address":string, "Start (Hz)":dbl, "Stop (Hz)":dbl, "Filter Order":i32, "Number of Points":i32, "Precision":u16, "Bandwidth (Hz)":dbl, "Averaging":u16, "Log Sweep":bool, "Demod":i32}
  T3 = typedef "cursor winow.ctl" = cluster{"left":dbl, "right ":dbl, "center":dbl, "window":dbl, "cursors":i32[], "relative":i32, "absolute":i32, "fixed vertical offset":dbl, "vertical offset":dbl, "skew":dbl, "default window frac":dbl, "kind":enum16{"symmetric", "skewed", "fancy"}, "skew.left":dbl, "skew.right":dbl, "Plot ref":refnum<vi>, "wing order":enum16{"forw", "back"}}
  T4 = enum32{"Everything", "Everything else", "even more "}
  T5 = cluster{"omega out":dbl[], "win omega out":dbl[]}
  T6 = typedef "lorentzian.ctl" = cluster{"Amplitude":dbl, "omega(0)":dbl, "Gamma":dbl, "phase":dbl, "Q":dbl, "Norm  Ampl":dbl, "z (inf)":cdb, "4corners":T7}
  T7 = typedef "circle corners.ctl" = cluster{"z (-pi/2)":cdb, "z(inf)":cdb, "z (pi/2)":cdb, "z center":cdb, "z(0)":cdb, "radius":dbl}
  T8 = typedef "eventvkey.ctl" = enum16{"ASCII", "Enter", "Return", "Shift", "Ctrl", "Alt", "Cmd", "Opt", "Caps", "NumLock", "Clear", "Break", "Up", "Down", "Left", "Right", "Insert", "Delete", "Home", "End", "PageUp", "PageDown", "Escape", "Help", "Pause", "ScrollLock", "F1", "F2", "F3", "F4", "F5", "F6", "F7", "F8", "F9", "F10", "F11", "F12", "F13", "F14", "F15", "F16", "F17", "F18", "F19", "F20", "F21", "F22", "F23", "F24", "Play", "VolumeUp", "VolumeDown", "Mute", "Two Byte Char"}
  T9 = typedef "peak -- parameters -- complex fit.ctl" = cluster{"main VI path":path, "scale factor":dbl, "# of grid points":i32, "parameters: wavepacket":T10, "span":dbl, "interference ?":enum16{"cp z center", "pm zcenter", "fancy"}, "filter method":T11}
  T10 = typedef "wavepacket.ctl" = cluster{"R":dbl, "wave number":dbl, "delta k":dbl, "radii vector":dbl[], "radial section":cdb[], "wave vector":dbl, "wavepacket is":bool}
  T11 = typedef "filter method control.ctl" = enum16{"four", "five", "one", "two", "three", "zero", "minus one", "minus two"}
  T12 = typedef "cursor window action.ctl" = enum16{"balance", "h. offset change", "cursor moves", "change center", "change window", "init", "check", "reset", "set y to middle", "idle", "-write all Y", "-write left.X", "-write center.X", "-write right.X", "-write all X", "-change center", "-change window", "-change skew", "-read cursor 2", "-read cursor 1", "-read cursor 0", "-read all cursors", "-reset", "-read plot scale", "-set y to middle", "-Q: center.Y is visible", "-Q: window is visible", "-parse center.Y", "-right left from center", "-left move", "-right move", "-set center.Y", "-empty", "-set cursors to default", "-check", "-write center.Y", "-copy cursor 1", "-copy cursor 0", "-copy cursor 2", "move right", "move left", "shrink", "broaden", "skew up", "skew down", "-write plot scale", "zoom X", "change cen&win", "zoom to all data"}
  T13 = typedef "plot refs -- filter related.ctl" = cluster{"Plot: complex plane - filter":refnum<vi>, "Plot: dz/domega":refnum<vi>, "Plot: fragment filter":refnum<vi>, "Plot: win omega":refnum<vi>, "Plot: phase":refnum<vi>, "Plot: phase around center":refnum<vi>, "Plot: complex plane":refnum<vi>, "Plot: fragment":refnum<vi>}
  T14 = typedef "KM_ControlHFLIcommand.ctl" = enum16{"Initialize", "Scan frequency"}
  T15 = typedef "KM_file -- read-write control.ctl" = enum16{"read", "write all", "append one line"}
  T16 = typedef "AdS_TempStatus.ctl" = cluster{"Sample Temp (K)":dbl, "VTI Temp (K)":dbl, "Sample Power (W)":dbl, "VTI Power (W)":dbl, "Temp Stable":bool}
  T17 = typedef "AdS_Status_Type.ctl" = cluster{"Sweep mode":u16, "Field (T)":dbl, "Upper sweep limit (T)":dbl, "Lower sweep limit (T)":dbl, "Switch heater":bool, "Voltage (V)":dbl, "Rate (T/min)":dbl, "Status":cluster{"Quench":bool, "Power Loss":bool, "Sweep":bool, "Standby":bool}, "PSU_Field (T)":dbl, "Interp. Field (T)":dbl, "PSU_Voltage (V)":dbl}
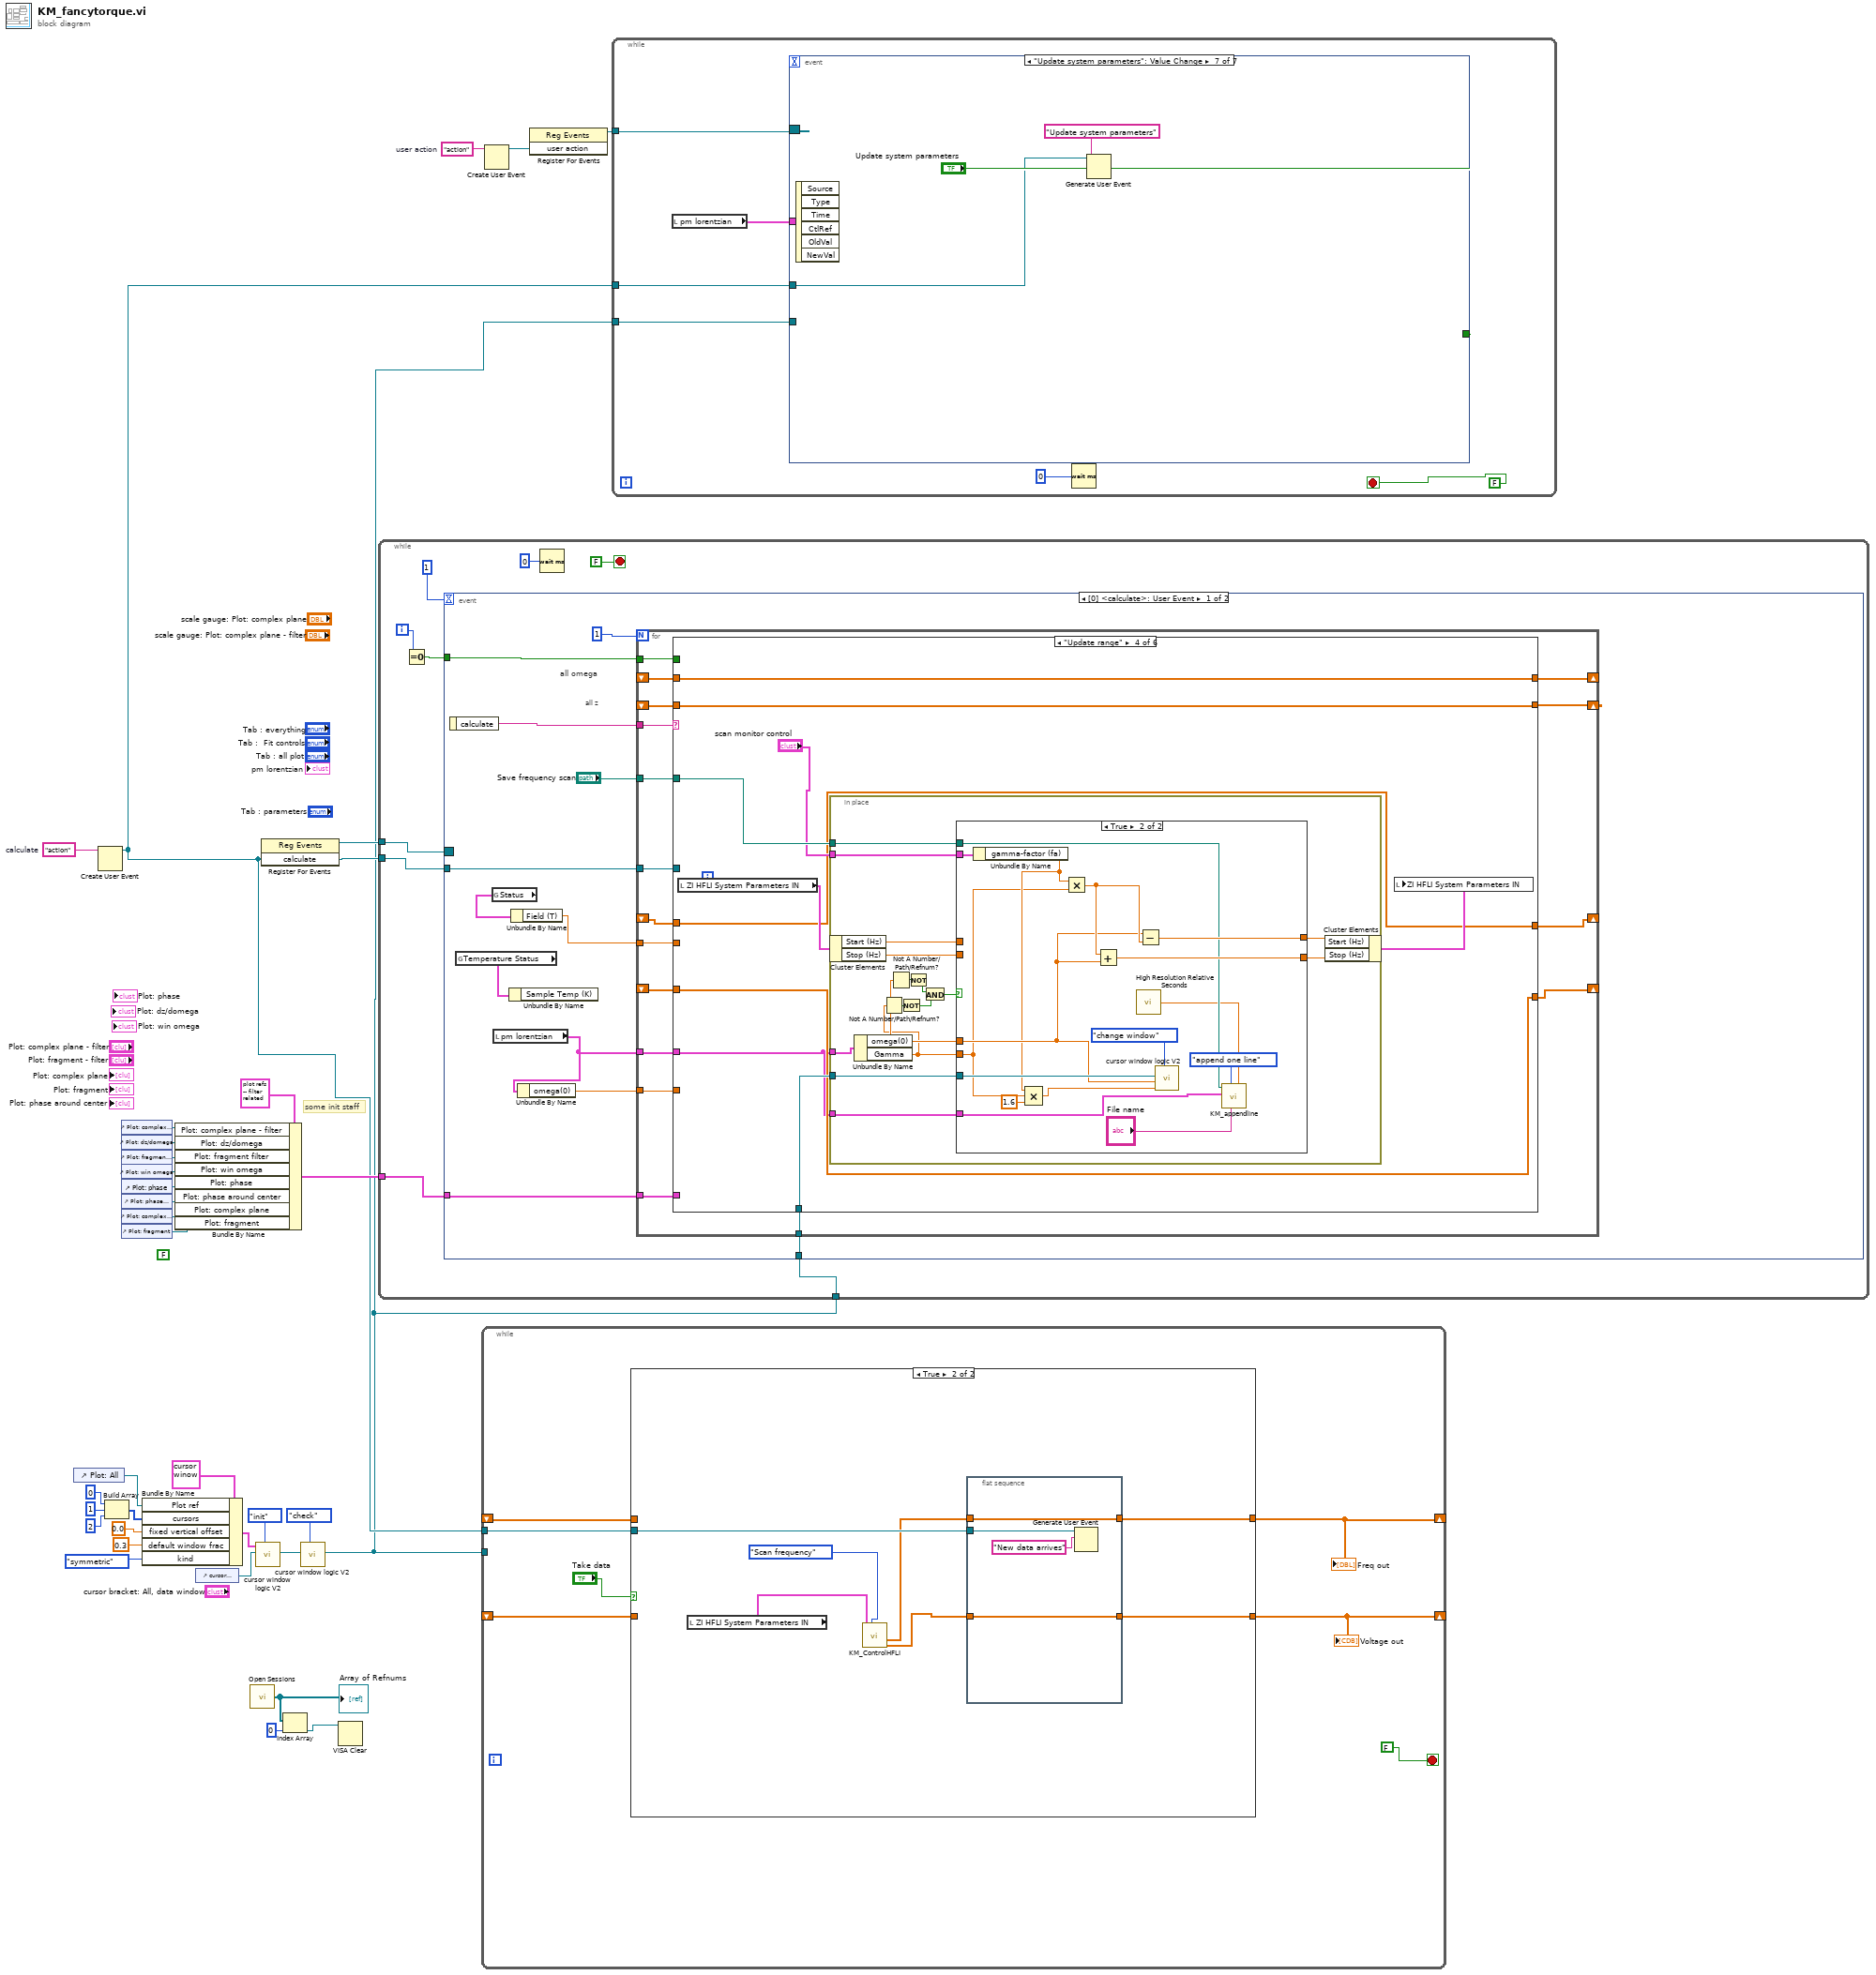
[diagram p0: block diagram]
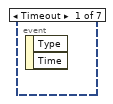
[diagram p3: hidden frame]
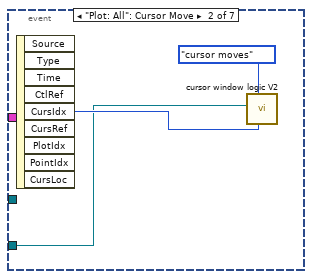
[diagram p4: hidden frame]
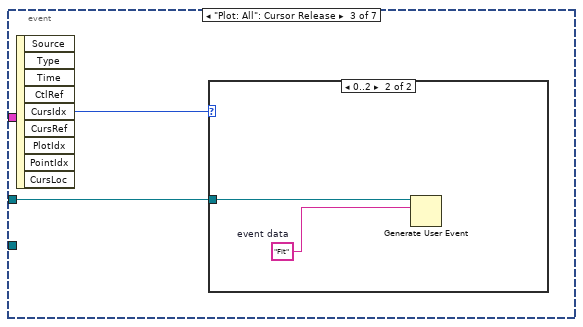
[diagram p5: hidden frame]
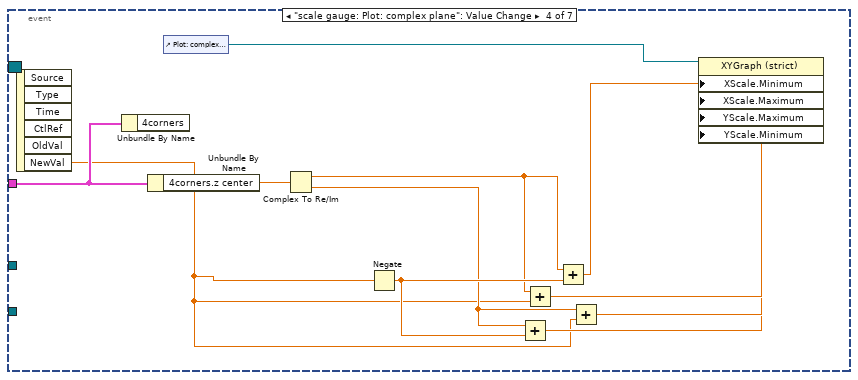
[diagram p7: hidden frame]
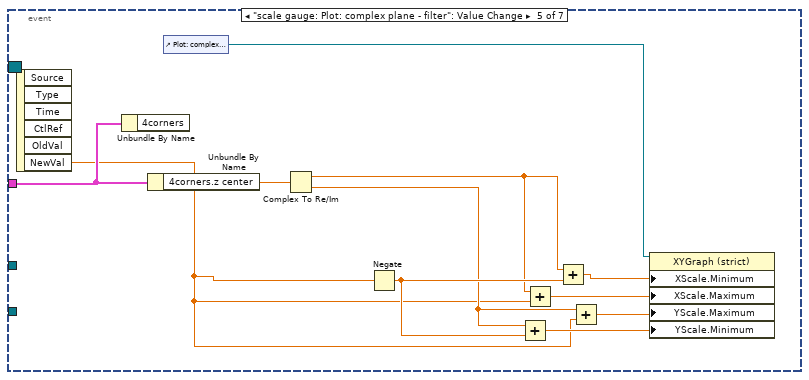
[diagram p8: hidden frame]
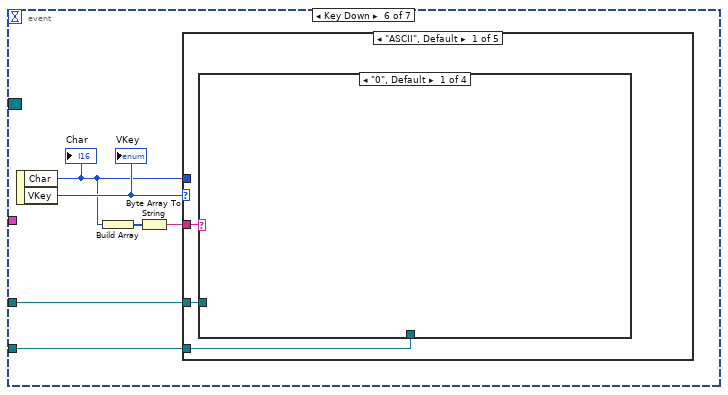
[diagram p9: hidden frame]
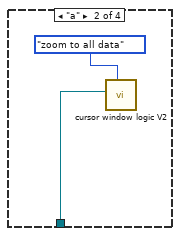
[diagram p10: hidden frame]
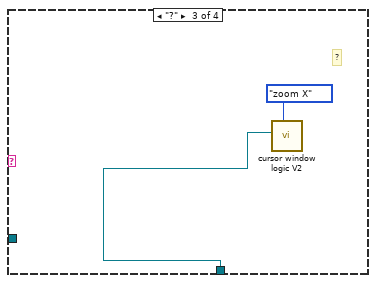
[diagram p11: hidden frame]
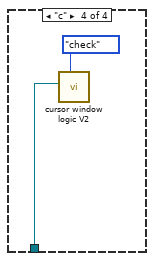
[diagram p12: hidden frame]
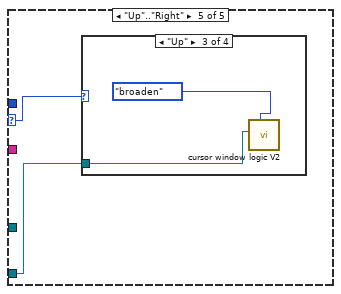
[diagram p16: hidden frame]
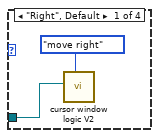
[diagram p17: hidden frame]
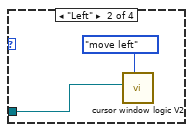
[diagram p18: hidden frame]
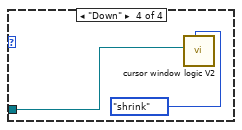
[diagram p19: hidden frame]
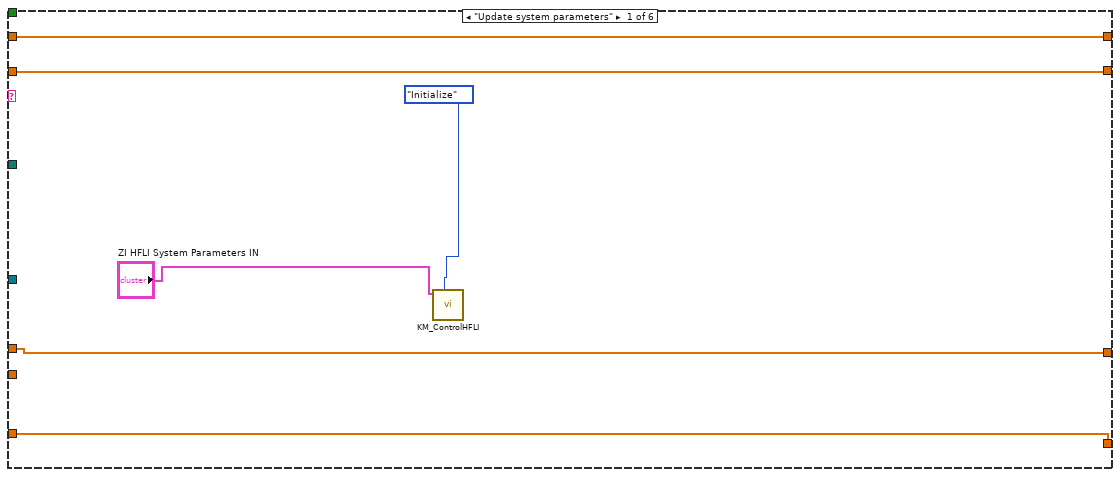
[diagram p20: hidden frame]
diagram:
  w31 = "action"  # user action
  w33 = "action"  # calculate
  (unwired) FALSE
  # "some init staff"
  n1 = control-ref of="Plot: All"() -> (w10:refnum<vi>)
  n2 = Create User Event(user event datatype=w33) -> (user event=w19:refnum<user-event>)  [unwired: 1 in, 1 out]
  n3 = Build Array(0, 1, 2) -> (w18:i32[])
  n4 = control-ref of="Plot: complex plane - filter"() -> (w28:refnum<vi>)
  n5 = control-ref of="Plot: dz/domega"() -> (w27:refnum<vi>)
  n6 = control-ref of="Plot: fragment - filter"() -> (w26:refnum<vi>)
  n7 = control-ref of="Plot: win omega"() -> (w25:refnum<vi>)
  n8 = control-ref of="Plot: phase"() -> (w24:refnum<vi>)
  n9 = control-ref of="Plot: phase around center"() -> (w22:refnum<vi>)
  n10 = control-ref of="Plot: complex plane"() -> (w21:refnum<vi>)
  n11 = control-ref of="Plot: fragment"() -> (w20:refnum<vi>)
  n12 = Bundle By Name(cluster=T3 {"left"=0.0, "right "=0.0, "center"=0.0, "window"=0.0, "cursors"=[], "relative"=0, "absolute"=0, "fixed vertical offset"=0.0, "vertical offset"=0.0, "skew"=0.0, "default window frac"=0.0, "kind"=enum."symmetric", "skew.left"=0.0, "skew.right"=0.0, "Plot ref"=refnum, "wing order"=enum."forw"} ("cursor bracket: All, data window"), "Plot ref"=w10, "cursors"=w18, "fixed vertical offset"=0.0, "default window frac"=0.3 ("fixed vertical offset"), "kind"=enum16{"symmetric", "skewed", "fancy"}."symmetric") -> (w9:T3)
  n13 = Bundle By Name(cluster=T13 {"Plot: complex plane - filter"=refnum, "Plot: dz/domega"=refnum, "Plot: fragment filter"=refnum, "Plot: win omega"=refnum, "Plot: phase"=refnum, "Plot: phase around center"=refnum, "Plot: complex plane"=refnum, "Plot: fragment"=refnum} ("plots: filter related"), "Plot: complex plane - filter"=w28, "Plot: dz/domega"=w27, "Plot: fragment filter"=w26, "Plot: win omega"=w25, "Plot: phase"=w24, "Plot: phase around center"=w22, "Plot: complex plane"=w21, "Plot: fragment"=w20) -> (w23:T13)
  n14 = control-ref of="cursor bracket: All, data window"() -> (w8:refnum<vi>)
  n15 = call <vilib>:"Open Sessions.vi"() -> ("Array of Refnums"=w1:refnum<visa-resource-name>[])  [unwired: 2 in]
  "Array of Refnums" <- w1
  n16 = call "cursor window logic V2.vi"("cursor window action"=cursor_window_action."init", "cursor window in"=w8, "cursor window init"=w9) -> ("cursor window out"=w6:refnum<vi>)  [unwired: 7 in, 1 out]
  n17 = register-events(w19) -> (reference out=w34:refnum<event-registration>)  [unwired: 2 in, 1 out]
  n18 = Index Array(array=w1, index=0) -> (element=w3:refnum<visa-resource-name>)
  n19 = call "cursor window logic V2.vi"("cursor window action"=cursor_window_action."check", "cursor window in"=w6) -> ("cursor window out"=w4:refnum<vi>)  [unwired: 8 in, 1 out]
  n20 = VISA Clear(VISA resource name=w3) -> ()  [unwired: 1 in, 2 out]
  n21 = while {
    tunnel: w34 -> [w43]
    tunnel: w19 -> [w41]
    tunnel: w23 -> [w37]
    tunnel: w4 -> [w35]
    i -> [w38]
    stop <- FALSE stop-if-true
    n22 = Equal To 0?(x=w38) -> (x = 0?=w36:bool)
    n23 = event shown="[0] <calculate>: User Event" {
      selector: w43 -> [_ _]
      dyn-events: _ -> [_ _]
      timeout: 1 -> [_ _]
      tunnel: w41 -> [w54 _]
      tunnel: w37 -> [w51 _]
      tunnel: w36 -> [w50 _]
      tunnel: w35 -> [w49 _]
      event User Event {
        # "all z"
        # "all omega"
        n24 = event-data() -> ("calculate"=w55:string)  [unwired: 1 in]
        n25 = global read "Magnet_August_der_Starke.vi" "Temperature Status"() -> (w48:T16)
        n26 = global read "Magnet_August_der_Starke.vi" "Status"() -> (w45:T17)
        n27 = local read "pm lorentzian"() -> (w46:T6)
        n28 = Unbundle By Name(w48) -> ()  [unwired: 1 out]
        n29 = Unbundle By Name(w45) -> ("Field (T)"=w44:dbl)
        n30 = Unbundle By Name(w46) -> ("omega(0)"=w47:dbl)
        n31 = for {
          N: 1 -> [_]
          tunnel: w55 -> [w72]
          tunnel: w54 -> [w71]
          shift-right: [w65] -> _
          shift-left: _ -> [w70]
          shift-right: [w64] -> _
          shift-left: _ -> [w69]
          tunnel: "Save frequency scan" -> [w68]
          tunnel: w51 -> [w67]
          tunnel: w50 -> [w66]
          tunnel: w49 -> [w63]
          tunnel: w47 -> [w62]
          tunnel: w46 -> [w61]
          shift-right: [w59] -> _
          shift-left: _ -> [w60]
          tunnel: w44 -> [w58]
          shift-right: [w57] -> _
          shift-left: _ -> [w56]
          n32 = case shown="\"Update range\"" w72 {
            tunnel: w71 -> [_ w87 _ _ _ _]
            tunnel: w70 -> [w78 _ w108 w118 w161 w171]
            tunnel: w69 -> [w77 _ w107 w117 w160 w170]
            tunnel: w68 -> [_ _ _ w113 _ _]
            tunnel: w67 -> [_ _ _ _ w162 _]
            tunnel: w66 -> [_ _ _ _ _ _]
            tunnel: [w78 w85 w108 w118 w161 w171] -> w65
            tunnel: [w77 w88 w107 w117 w160 w170] -> w64
            tunnel: w63 -> [_ _ _ w114 w157 _]
            tunnel: w62 -> [_ _ w104 _ _ _]
            tunnel: w61 -> [_ _ _ w109 _ _]
            tunnel: w60 -> [w74 w79 w106 w111 w154 w169]
            tunnel: [w74 w79 w102 w111 w154 w169] -> w59
            tunnel: w58 -> [_ _ w105 _ _ _]
            tunnel: [w73 w81 w101 w110 w153 w168] -> w57
            tunnel: w56 -> [w73 w81 w103 w110 w153 w168]
            frame "Update system parameters" {
              n33 = call "KM_ControlHFLI.vi"("Control HFLI command"=KM_ControlHFLIcommand."Initialize", "ZI HFLI System Parameters IN"="ZI HFLI System Parameters IN") -> ()  [unwired: 4 in, 3 out]
            }
            frame "New data arrives" {
              n34 = local read "Voltage out"() -> (w88:cdb[])
              n35 = local read "Freq out"() -> (w85:dbl[])
              n36 = Complex To Re/Im(x + iy=w88) -> (x=w91:dbl[], y=w90:dbl[])
              n37 = Bundle("Freq out"=w85, w91) -> (w92:cluster{"Freq out":dbl[], dbl[]})  [unwired: 1 in]
              n38 = Bundle("Freq out"=w85, w90) -> (w89:cluster{"Freq out":dbl[], dbl[]})  [unwired: 1 in]
              n39 = Build Array(w92, w89) -> (→"Plot: All":cluster{"Freq out":dbl[], dbl[]}[])
              n40 = Generate User Event(user event=w87, event data cluster="Fit" ("event data")) -> (user event out=w83:refnum<user-event>)  [unwired: 2 in, 1 out]
              n41 = case shown="True" "Update range" {
                tunnel: w83 -> [w94 w96]
                tunnel: [w94 w95] -> w82
                frame False {
                }
                frame True {
                  n42 = Generate User Event(user event=w96, event data cluster="Update range" ("event data")) -> (user event out=w95:refnum<user-event>)  [unwired: 2 in, 1 out]
                }
              }
              n43 = case shown="False" "Plot frequency shift" {
                tunnel: w82 -> [_ w98]
                frame False {
                }
                frame True {
                  n44 = Generate User Event(user event=w98, event data cluster="Plot frequency shift" ("event data")) -> ()  [unwired: 2 in, 2 out]
                }
              }
            }
            frame "Plot frequency shift" {
              n45 = Build Array (concatenate)(w103, w104) -> (w101:dbl[])
              n46 = Build Array (concatenate)(w106, w105) -> (w102:dbl[])
              n47 = Bundle(w102, w101) -> (→"Plot: freq vs T":cluster{dbl[], dbl[]})  [unwired: 1 in]
            }
            frame "Update range" {
              n48 = local read "ZI HFLI System Parameters IN"() -> (w116:T2)
              n49 = in-place {
                in-place-border: "scan monitor control" -> [w134]
                in-place-border: w114 -> [w122]
                in-place-border: w113 -> [w121]
                in-place-border: w109 -> [w120]
                in-place-border: w109 -> [w119]
                n50 = in-place-cluster #1(w116) -> ("Start (Hz)"=w124:dbl, "Stop (Hz)"=w123:dbl)
                n51 = Unbundle By Name(w120) -> ("omega(0)"=w131:dbl, "Gamma"=w126:dbl)
                n52 = Not A Number/Path/Refnum?(number/path/refnum=w126) -> (NaN/Path/Refnum?=w127:bool)
                n53 = Not A Number/Path/Refnum?(number/path/refnum=w131) -> (NaN/Path/Refnum?=w129:bool)
                n54 = Not(x=w127) -> (.not. x?=w125:bool)
                n55 = Not(x=w129) -> (.not. x?=w128:bool)
                n56 = And(x=w128, y=w125) -> (x .and. y?=w130:bool)
                n57 = case shown="True" w130 {
                  tunnel: w134 -> [_ w152]
                  tunnel: [w135 w151] -> w133
                  tunnel: w126 -> [_ w144]
                  tunnel: w131 -> [_ w146]
                  tunnel: [w136 w149] -> w132
                  tunnel: w124 -> [w136 _]
                  tunnel: w123 -> [w135 _]
                  tunnel: w122 -> [_ w147]
                  tunnel: w121 -> [_ w140]
                  tunnel: w119 -> [_ w137]
                  frame False {
                  }
                  frame True {
                    n58 = Unbundle By Name(w152) -> ("gamma-factor (fa)"=w145:dbl)
                    n59 = Compound Arithmetic op=MULTIPLY(w145, w144, 1.6 ("value")) -> (w142:dbl)
                    n60 = Multiply(x=w145, y=w144) -> (x*y=w150:dbl)
                    n61 = Add(x=w150, y=w146) -> (x+y=w151:dbl)
                    n62 = call <vilib>:"High Resolution Relative Seconds.vi"() -> ("relative seconds"=w138:dbl)
                    n63 = Subtract(x=w146, y=w150) -> (x-y=w149:dbl)
                    n64 = call "cursor window logic V2.vi"("cursor window action"=cursor_window_action."change window", "window"=w142, "center"=w146, "cursor window in"=w147) -> ()  [unwired: 6 in, 2 out]
                    n65 = call "KM_appendline.vi"("Time (s)"=w138, "name or relative path"="File name", "read/write control"=KM_file_--_read-write_control."append one line", "pm lorentzian"=w137, "Save frequency scan"=w140) -> ()  [unwired: 7 in]
                  }
                }
                n66 = in-place-cluster #1("Start (Hz)"=w132, "Stop (Hz)"=w133) -> (w115:T2)
              }
              n67 = local write "ZI HFLI System Parameters IN"(w115) -> ()
            }
            frame "Fit" {
              n68 = call "cursor window logic V2.vi"("cursor window action"=cursor_window_action."check", "cursor window in"=w157) -> ("cursor window out"=w159:T3)  [unwired: 8 in, 1 out]
              n69 = call "acquire cursor window data.vi"("z in"=w160, "omega in"=w161, "cursor window"=w159) -> ("z out"=w155:cdb[], "omega  out"=w156:dbl[])  [unwired: 4 in, 3 out]
              n70 = call "KM_peak -- find -- pm - V1.vi"("omega in"=w156, "z in"=w155, "parameters: complex fit"="parameters: complex fit", "plots: filter related"=w162, "plot staff ?"="plot staff", "just guess?"="use fast fit?", "subtract linear BG"=FALSE) -> ("pm lorentzian"=w163:T6)  [unwired: 10 in, 2 out]
              n71 = local write "pm lorentzian"(w163) -> ()
            }
            frame "Void", Default {
            }
          }
        }
      }
      event Timeout {
        n72 = event-data() -> ()  [unwired: 1 in, 2 out]
      }
    }
    n73 = Wait (ms)(milliseconds to wait=u32 0) -> ()  [unwired: 1 out]
  }
  n74 = while {
    shift-right: [w178] -> _
    shift-left: _ -> [w176]
    shift-right: [w177] -> _
    shift-left: _ -> [w175]
    tunnel: w19 -> [w174]
    tunnel: w4 -> [_]
    stop <- FALSE stop-if-true
    n75 = case shown="True" "Take data" {
      tunnel: [w180 w186] -> w178
      tunnel: [w179 w185] -> w177
      tunnel: w176 -> [w180 _]
      tunnel: w175 -> [w179 _]
      tunnel: w174 -> [_ w187]
      frame False {
      }
      frame True {
        n76 = local read "ZI HFLI System Parameters IN"() -> (w181:T2)
        n77 = call "KM_ControlHFLI.vi"("Control HFLI command"=KM_ControlHFLIcommand."Scan frequency", "ZI HFLI System Parameters IN"=w181) -> ("Voltage out"=w183:cdb[], "Freq out"=w184:dbl[])  [unwired: 4 in, 1 out]
        n78 = flat-sequence {
          tunnel: w184 -> [w191]
          tunnel: [w191] -> w186
          tunnel: w183 -> [w190]
          tunnel: [w190] -> w185
          tunnel: w187 -> [w188]
          frame #0 {
            n79 = Generate User Event(user event=w188, event data cluster="New data arrives" ("event data")) -> ()  [unwired: 2 in, 2 out]
          }
        }
      }
    }
    "Freq out" <- w178
    "Voltage out" <- w177
  }
  n80 = Create User Event(user event datatype=w31) -> (user event=w30:refnum<user-event>)  [unwired: 1 in, 1 out]
  n81 = register-events(w30) -> (reference out=w32:refnum<event-registration>)  [unwired: 2 in, 1 out]
  n82 = while {
    tunnel: w32 -> [w197]
    tunnel: w19 -> [w195]
    tunnel: w4 -> [w194]
    stop <- FALSE stop-if-true
    n83 = local read "pm lorentzian"() -> (w193:T6)
    n84 = event shown="[6] \"Update system parameters\": Value Change" {
      selector: w197 -> [_ _ _ _ _ _ _]
      dyn-events: _ -> [_ _ _ _ _ _ _]
      timeout: _ -> [_ _ _ _ _ _ _]
      tunnel: w195 -> [_ _ w202 _ _ w231 w252]
      tunnel: [_ _ _ _ _ _ "Update system parameters"] -> _
      tunnel: w194 -> [_ w199 _ _ _ w227 _]
      tunnel: w193 -> [_ _ _ w207 w218 _ _]
      event Timeout {
        n85 = event-data() -> ()  [unwired: 1 in, 2 out]
      }
      event "Plot: All": Cursor Move {
        n86 = event-data() -> ("CursIdx"=w200:i32)  [unwired: 1 in, 8 out]
        n87 = call "cursor window logic V2.vi"("CursIdx"=w200, "cursor window action"=cursor_window_action."cursor moves", "cursor window in"=w199) -> ()  [unwired: 7 in, 2 out]
      }
      event "Plot: All": Cursor Release {
        n88 = event-data() -> ("CursIdx"=w201:i32)  [unwired: 1 in, 8 out]
        n89 = case shown="0..2" w201 {
          tunnel: w202 -> [_ w203]
          frame 3, Default {
          }
          frame 0..2 {
            w204 = "Fit"  # event data
            n90 = Generate User Event(user event=w203, event data cluster=w204) -> ()  [unwired: 2 in, 2 out]
          }
        }
      }
      event "scale gauge: Plot: complex plane": Value Change {
        n91 = event-data() -> ("NewVal"=w206:dbl)  [unwired: 1 in, 5 out]
        n92 = Unbundle By Name(w207) -> ()  [unwired: 1 out]
        n93 = Unbundle By Name(w207) -> ("4corners.z center"=w208:cdb)
        n94 = control-ref of="Plot: complex plane"() -> (w205:refnum<vi>)
        n95 = Complex To Re/Im(x + iy=w208) -> (x=w209:dbl, y=w210:dbl)
        n96 = Negate(x=w206) -> (-x=w215:dbl)
        n97 = Add(x=w210, y=w215) -> (x+y=w211:dbl)
        n98 = Add(x=w209, y=w206) -> (x+y=w213:dbl)
        n99 = Add(x=w209, y=w215) -> (x+y=w214:dbl)
        n100 = Add(x=w210, y=w206) -> (x+y=w212:dbl)
        n101 = property on="Property Node" class="XYGraph (strict)"(reference=w205, "XScale.Minimum"=w214, "XScale.Maximum"=w213, "YScale.Maximum"=w212, "YScale.Minimum"=w211) -> ()  [unwired: 1 in, 2 out]
      }
      event "scale gauge: Plot: complex plane - filter": Value Change {
        n102 = event-data() -> ("NewVal"=w217:dbl)  [unwired: 1 in, 5 out]
        n103 = Unbundle By Name(w218) -> ()  [unwired: 1 out]
        n104 = Unbundle By Name(w218) -> ("4corners.z center"=w219:cdb)
        n105 = control-ref of="Plot: complex plane - filter"() -> (w216:refnum<vi>)
        n106 = Complex To Re/Im(x + iy=w219) -> (x=w220:dbl, y=w221:dbl)
        n107 = Negate(x=w217) -> (-x=w226:dbl)
        n108 = Add(x=w221, y=w226) -> (x+y=w222:dbl)
        n109 = Add(x=w220, y=w217) -> (x+y=w224:dbl)
        n110 = Add(x=w220, y=w226) -> (x+y=w225:dbl)
        n111 = Add(x=w221, y=w217) -> (x+y=w223:dbl)
        n112 = property on="Property Node" class="XYGraph (strict)"(reference=w216, "XScale.Minimum"=w225, "XScale.Maximum"=w224, "YScale.Maximum"=w223, "YScale.Minimum"=w222) -> ()  [unwired: 1 in, 2 out]
      }
      event Key Down {
        n113 = event-data() -> ("Char"=w229:i16, "VKey"=w232:T8)  [unwired: 1 in]
        "Char" <- w229
        "VKey" <- w232
        n114 = Build Array(w229) -> (w230:i16[])
        n115 = Byte Array To String(unsigned byte array=w230) -> (string=w228:string)
        n116 = case shown="\"ASCII\", Default" w232 {
          selector: w232 -> [_ _ _ _ w242]
          tunnel: w229 -> [_ _ _ _ _]
          tunnel: w231 -> [w235 _ _ _ _]
          tunnel: w228 -> [w234 _ _ _ _]
          tunnel: w227 -> [w233 _ _ _ w243]
          frame "ASCII", Default {
            n117 = case shown="\"0\", Default" w234 {
              tunnel: w235 -> [_ _ _ _]
              tunnel: w233 -> [_ w236 w238 w240]
              frame "0", Default {
              }
              frame "a" {
                n118 = call "cursor window logic V2.vi"("cursor window action"=cursor_window_action."zoom to all data", "cursor window in"=w236) -> ()  [unwired: 8 in, 2 out]
              }
              frame "?" {
                # "?"
                n119 = call "cursor window logic V2.vi"("cursor window action"=cursor_window_action."zoom X", "cursor window in"=w238) -> ()  [unwired: 8 in, 2 out]
              }
              frame "c" {
                n120 = call "cursor window logic V2.vi"("cursor window action"=cursor_window_action."check", "cursor window in"=w240) -> ()  [unwired: 8 in, 2 out]
              }
            }
          }
          frame "Escape" {
          }
          frame "PageUp" {
          }
          frame "PageDown" {
          }
          frame "Up".."Right" {
            n121 = case shown="\"Up\"" w242 {
              tunnel: w243 -> [w244 w246 w248 w251]
              frame "Right", Default {
                n122 = call "cursor window logic V2.vi"("cursor window action"=cursor_window_action."move right", "cursor window in"=w244) -> ()  [unwired: 8 in, 2 out]
              }
              frame "Left" {
                n123 = call "cursor window logic V2.vi"("cursor window action"=cursor_window_action."move left", "cursor window in"=w246) -> ()  [unwired: 8 in, 2 out]
              }
              frame "Up" {
                n124 = call "cursor window logic V2.vi"("cursor window action"=cursor_window_action."broaden", "cursor window in"=w248) -> ()  [unwired: 8 in, 2 out]
              }
              frame "Down" {
                n125 = call "cursor window logic V2.vi"("cursor window action"=cursor_window_action."shrink", "cursor window in"=w251) -> ()  [unwired: 8 in, 2 out]
              }
            }
          }
        }
      }
      event "Update system parameters": Value Change {
        n126 = event-data() -> ()  [unwired: 1 in, 6 out]
        n127 = Generate User Event(user event=w252, event data cluster="Update system parameters" ("event data")) -> ()  [unwired: 2 in, 2 out]
      }
    }
    n128 = Wait (ms)(milliseconds to wait=u32 0) -> ()  [unwired: 1 out]
  }
